vi "AddRecordFile.vi"(8 "에러 입력":errorcluster, 10 "LabTime":string, 11 "파일 경로(대화 상자 사용)":path=path "C:/Users/jinbeom/Desktop/data.txt") -> (0 "에러 출력":errorcluster, 3 "경로":path)   [LabVIEW 2017]
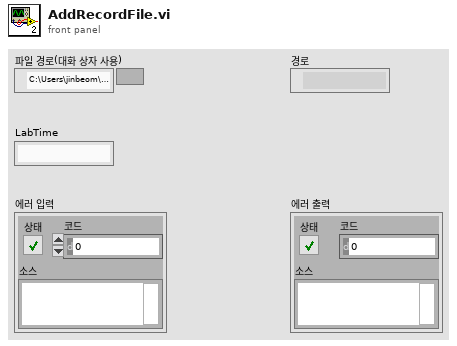
[diagram p1: front panel]
types:
  T1 = enum16{"open", "replace", "create", "open or create", "replace or create", "replace or create with confirmation"}
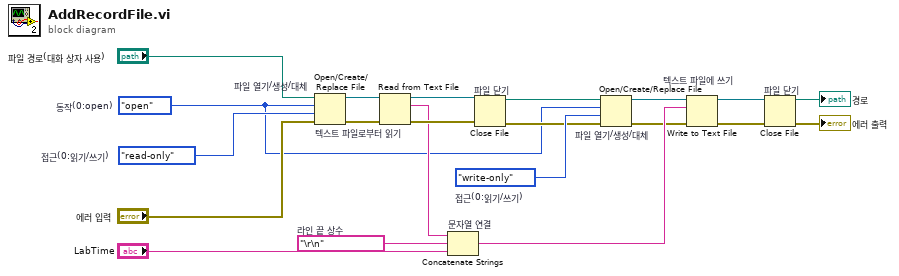
[diagram p0: block diagram]
diagram:
  w16 = "\r\n"  # 라인 끝 상수
  w18 = enum16{"read/write", "read-only", "write-only"}."write-only"  # 접근(0:읽기/쓰기)
  w21 = enum16{"read/write", "read-only", "write-only"}."read-only"  # 접근(0:읽기/쓰기)
  w3 = T1."open"  # 동작(0:open)
  n1 = Open/Create/Replace File "파일 열기/생성/대체"(file path (use dialog)="파일 경로(대화 상자 사용)", error in="에러 입력", operation (0:open)=w3, access (0:read/write)=w21) -> (refnum out=w19:refnum<file>, error out=w14:errorcluster)  [unwired: 2 in, 1 out]
  n2 = Read from Text File "텍스트 파일로부터 읽기"(file (use dialog)=w19, error in=w14) -> (refnum out=w12:refnum<file>, text=w8:string, error out=w11:errorcluster)  [unwired: 2 in, 1 out]
  n3 = Concatenate Strings "문자열 연결"(w8, w16, "LabTime") -> (w15:string)
  n4 = Close File "파일 닫기"(refnum=w12, error in=w11) -> (path=w10:path, error out=w9:errorcluster)
  n5 = Open/Create/Replace File "파일 열기/생성/대체"(file path (use dialog)=w10, error in=w9, operation (0:open)=w3, access (0:read/write)=w18) -> (refnum out=w17:refnum<file>, error out=w13:errorcluster)  [unwired: 2 in, 1 out]
  n6 = Write to Text File "텍스트 파일에 쓰기"(file (use dialog)=w17, text=w15, error in=w13) -> (refnum out=w7:refnum<file>, error out=w6:errorcluster)  [unwired: 1 in, 1 out]
  n7 = Close File "파일 닫기"(refnum=w7, error in=w6) -> (path=→"경로":path, error out=→"에러 출력":errorcluster)
